vi "array2str.vi"(1 "array in":dbl[](array[numeric]) format="%.2f") -> (0 "string out":string)   [LabVIEW 2017]
doc: "Transforms an array into a string of the numbers \nDelimiter is a space"
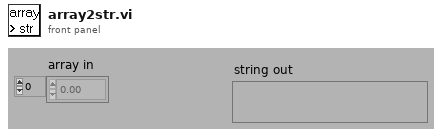
[diagram p1: front panel]
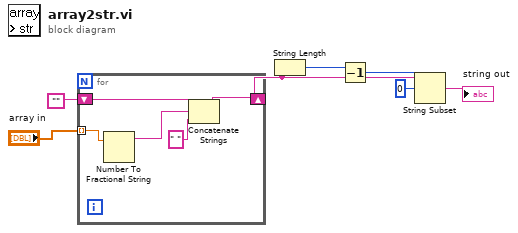
[diagram p0: block diagram]
diagram:
  n1 = for {
    tunnel: "array in" -> [w12] mode=indexing
    shift-right: [w9] -> w4
    shift-left: "" -> [w11]
    n2 = Number To Fractional String(number=w12) -> (F-format string=w10:string)  [unwired: 3 in]
    n3 = Concatenate Strings(w11, w10, " ") -> (w9:string)
  }
  n4 = String Length(string=w4) -> (length=w2:i32)
  n5 = Decrement(x=w2) -> (x-1=w1:i32)
  n6 = String Subset(string=w4, offset (0)=0, length (rest)=w1) -> (substring=→"string out":string)
